vi "PID_controller_15.vi"() -> ()   [LabVIEW 2011]
panel:
  out "do_tune":bool
  in  "Tune":bool
  out "Temp Set Point (torr)":dbl
  in  "stop":bool
  out "fit":cluster{"element":dbl, "Value":dbl}[](array[cluster])
  out "err_avg":dbl
  out "Setpoint":string
  in  "Ks":dbl
  out "dt(s)":dbl
  out "windup error":dbl
  out "tPrev":dbl
  out "target value":dbl
  out "error(t-t0)":cluster{dbl, "Value":dbl}[](array[cluster])
  out "error":dbl
  out "tStart(s)":dbl
  out "S00":dbl
  out "S10":dbl
  out "S20":dbl
  out "S11":dbl
  out "S01":dbl
  out "weight":dbl[](array[numeric])
  in  "# of points to watch":i32
  in  "tSmooth(s)":dbl=-1.0
  out "t0":dbl
  out "error(t)":cluster{dbl, "Value":dbl}[](array[cluster])
  out "error out":errorcluster
  out "first":bool=TRUE
  out "XY Graph":T1(graph)
  out "current value":dbl
  in  "Period (s)":dbl
  out "dValue":dbl
  out "derivative":dbl
  out "integral":dbl
  out "Angle (deg)":dbl
  in  "Kd":dbl
  in  "Ki":dbl
  in  "Kp":dbl
  out "Current P (torr)":dbl
  in  "Set Point (torr)":dbl
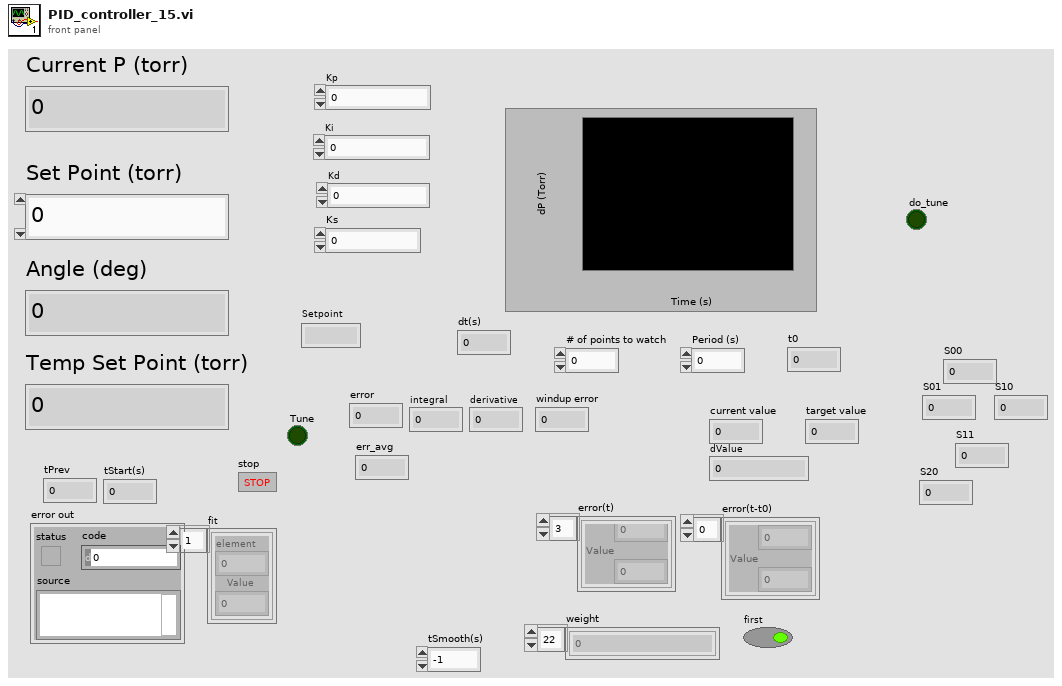
[diagram p1: front panel]
types:
  T1 = cluster{"Value":cluster{"element":dbl, "Value":dbl}[]}[]
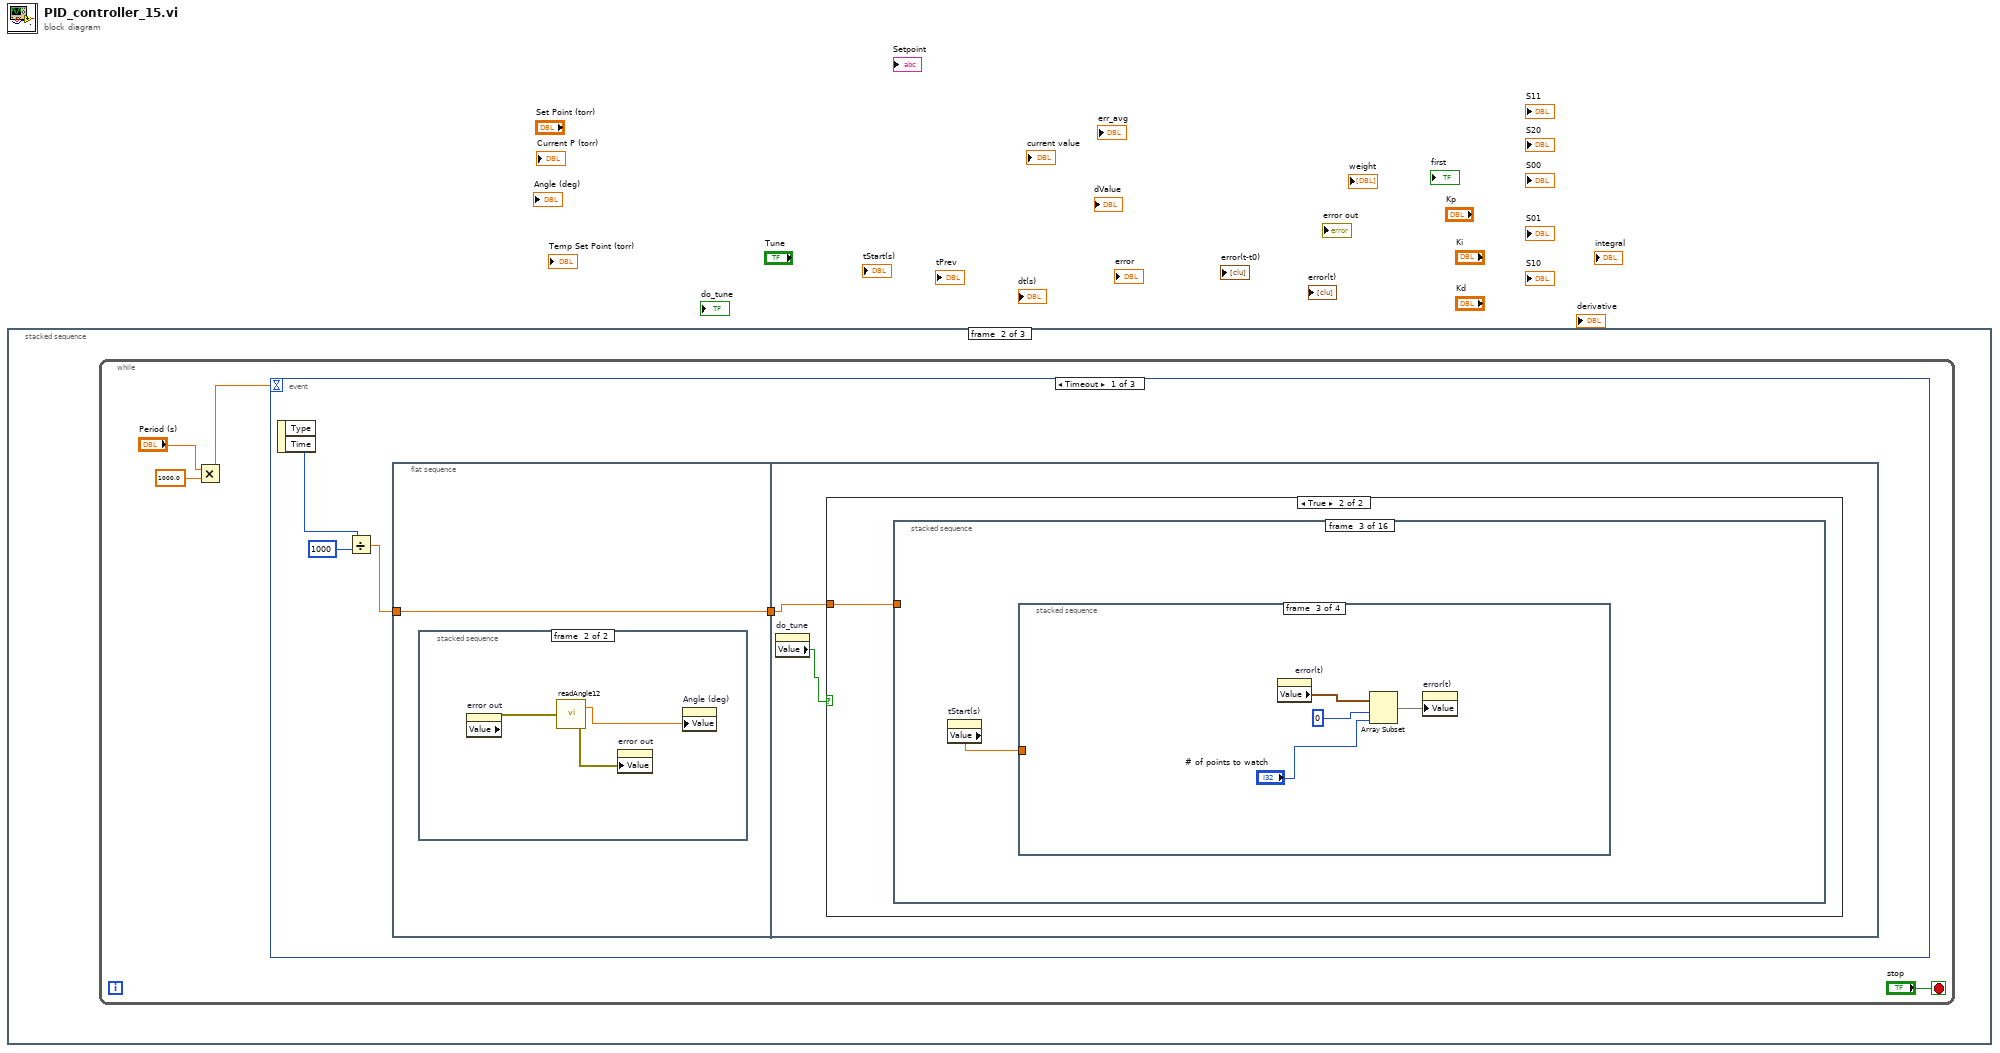
[diagram p0: block diagram]
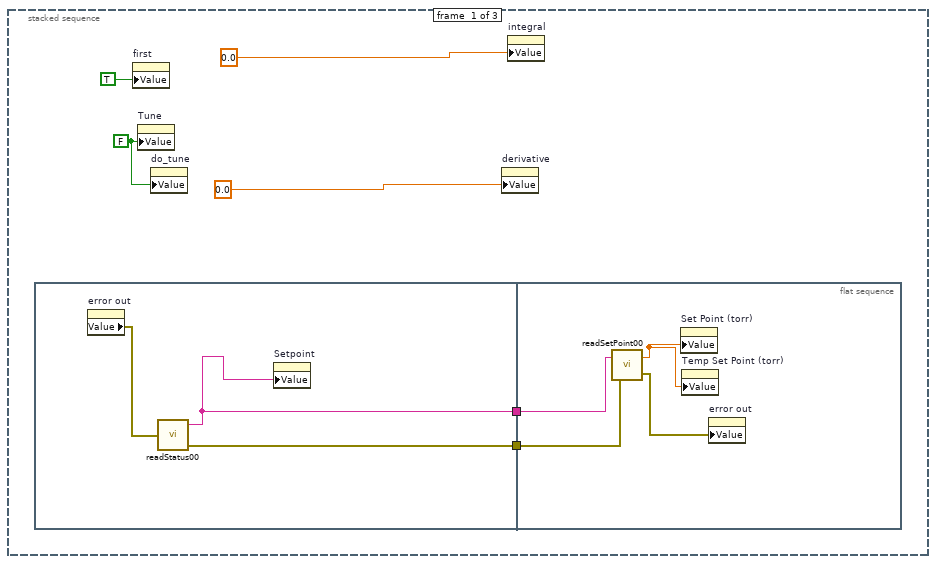
[diagram p2: hidden frame]
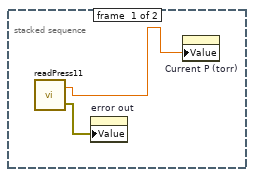
[diagram p3: hidden frame]
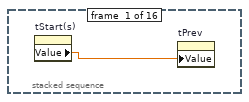
[diagram p5: hidden frame]
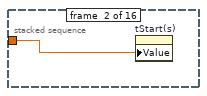
[diagram p6: hidden frame]
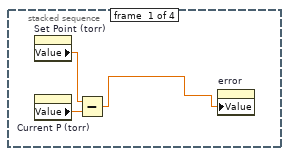
[diagram p7: hidden frame]
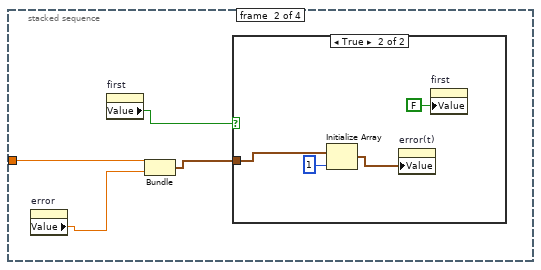
[diagram p8: hidden frame]
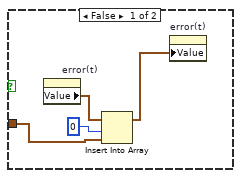
[diagram p9: hidden frame]
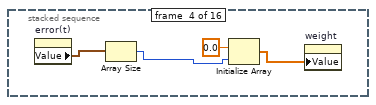
[diagram p11: hidden frame]
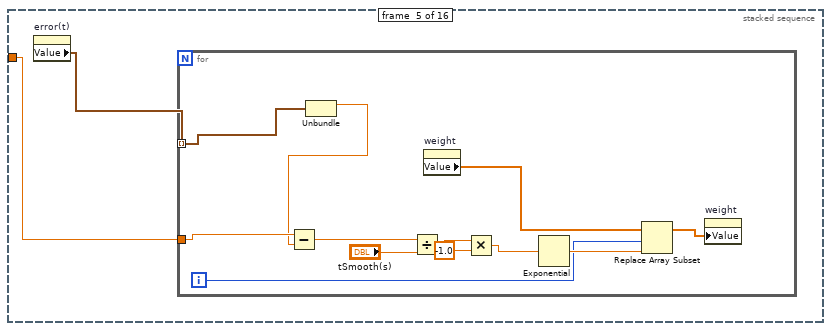
[diagram p12: hidden frame]
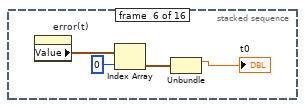
[diagram p13: hidden frame]
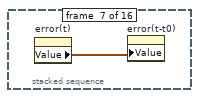
[diagram p14: hidden frame]
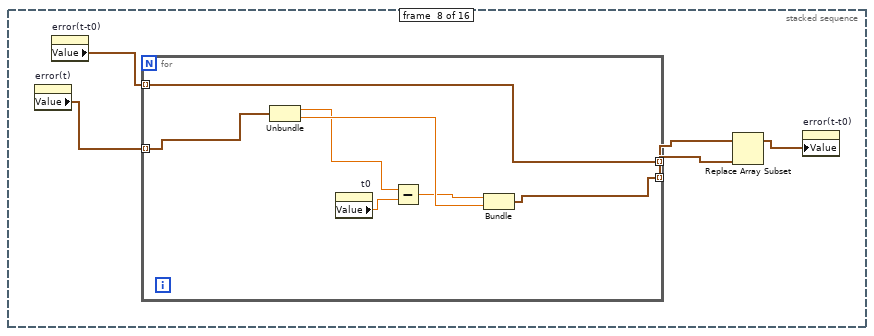
[diagram p15: hidden frame]
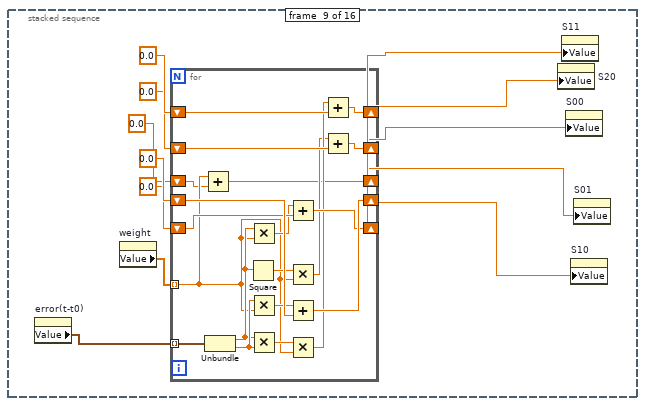
[diagram p16: hidden frame]
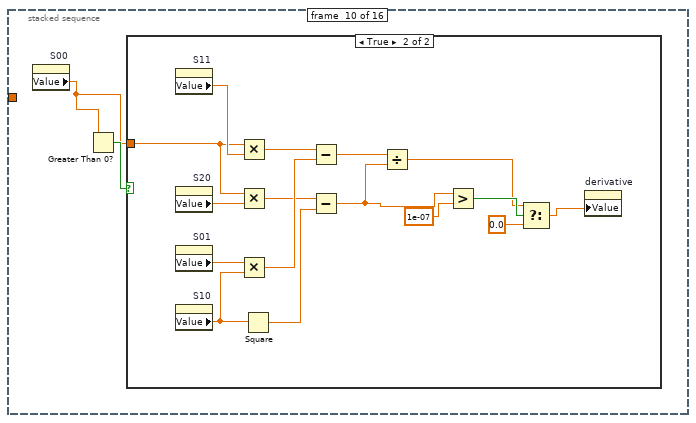
[diagram p17: hidden frame]
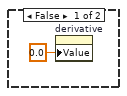
[diagram p18: hidden frame]
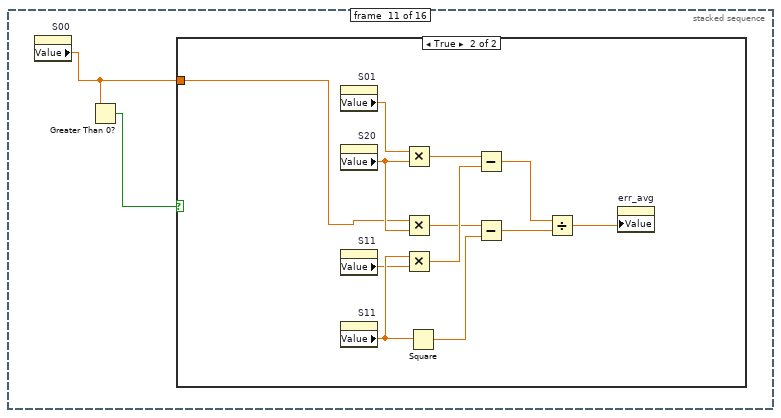
[diagram p19: hidden frame]
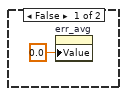
[diagram p20: hidden frame]
diagram:
  n1 = stacked-sequence {
    frame #0 {
      w1 = FALSE ("Tune")
      n2 = flat-sequence {
        tunnel: [w8] -> w3
        tunnel: [w7] -> w2
        tunnel: w3 -> [w13]
        tunnel: w2 -> [w12]
        frame #0 {
          n3 = property on="error out" class="Clust (strict)"() -> ("Value"=w9:errorcluster)  [unwired: 2 in, 2 out]
          n4 = call "readStatus00.vi"("error in"=w9) -> ("Setpoint"=w8:string, "error out"=w7:errorcluster)  [unwired: 1 out]
          n5 = property on="Setpoint" class="Str"("Value"=w8) -> ()  [unwired: 2 in, 2 out]
        }
        frame #1 {
          n6 = call "readSetPoint00.vi"("error in"=w12, "Setpoint"=w13) -> ("error out"=w11:errorcluster, "P"=w10:dbl)
          n7 = property on="Set Point (torr)" class="DigNum (strict)"("Value"=w10) -> ()  [unwired: 2 in, 2 out]
          n8 = property on="Temp Set Point (torr)" class="DigNum (strict)"("Value"=w10) -> ()  [unwired: 2 in, 2 out]
          n9 = property on="error out" class="Clust (strict)"("Value"=w11) -> ()  [unwired: 2 in, 2 out]
        }
      }
      n10 = property on="first" class="Bool (strict)"("Value"=TRUE ("first")) -> ()  [unwired: 2 in, 2 out]
      n11 = property on="Tune" class="Bool (strict)"("Value"=w1) -> ()  [unwired: 2 in, 2 out]
      n12 = property on="do_tune" class="Bool (strict)"("Value"=w1) -> ()  [unwired: 2 in, 2 out]
      n13 = property on="derivative" class="DigNum (strict)"("Value"=0.0 ("derivative")) -> ()  [unwired: 2 in, 2 out]
      n14 = property on="integral" class="DigNum (strict)"("Value"=0.0 ("integral")) -> ()  [unwired: 2 in, 2 out]
    }
    frame #1 {
      n15 = while {
        stop <- "stop" stop-if-true
        n16 = Multiply(x="Period (s)", y=1000.0) -> (x*y=w15:dbl)
        n17 = event shown="[0] Timeout" {
          selector: _ -> [_ _ _]
          dyn-events: _ -> [_ _ _]
          timeout: w15 -> [_ _ _]
          event Timeout {
            n18 = event-data() -> ("Time"=w21:u32)  [unwired: 1 in, 1 out]
            n19 = Divide(x=w21, y=u32 1000) -> (x/y=w19:dbl)
            n20 = flat-sequence {
              tunnel: w19 -> [w22]
              tunnel: [w22] -> w18
              tunnel: w18 -> [w29]
              frame #0 {
                n21 = stacked-sequence {
                  frame #0 {
                    n22 = call "readPress11.vi"() -> ("P"=w24:dbl, "error out"=w23:errorcluster)  [unwired: 1 in]
                    n23 = property on="error out" class="Clust (strict)"("Value"=w23) -> ()  [unwired: 2 in, 2 out]
                    n24 = property on="Current P (torr)" class="DigNum (strict)"("Value"=w24) -> ()  [unwired: 2 in, 2 out]
                  }
                  frame #1 {
                    n25 = property on="error out" class="Clust (strict)"() -> ("Value"=w26:errorcluster)  [unwired: 2 in, 2 out]
                    n26 = call "readAngle12.vi"("error in"=w26) -> ("angle"=w27:dbl, "error out"=w25:errorcluster)
                    n27 = property on="error out" class="Clust (strict)"("Value"=w25) -> ()  [unwired: 2 in, 2 out]
                    n28 = property on="Angle (deg)" class="DigNum (strict)"("Value"=w27) -> ()  [unwired: 2 in, 2 out]
                  }
                }
              }
              frame #1 {
                n29 = property on="do_tune" class="Bool (strict)"() -> ("Value"=w28:bool)  [unwired: 2 in, 2 out]
                n30 = case shown="True" w28 {
                  tunnel: w29 -> [_ w30]
                  frame False {
                  }
                  frame True {
                    n31 = stacked-sequence {
                      tunnel: w30 -> [_ w32 _ _ w57 _ _ _ _ _ _ _ _ _ _ _]
                      frame #0 {
                        n32 = property on="tStart(s)" class="DigNum (strict)"() -> ("Value"=w31:dbl)  [unwired: 2 in, 2 out]
                        n33 = property on="tPrev" class="DigNum (strict)"("Value"=w31) -> ()  [unwired: 2 in, 2 out]
                      }
                      frame #1 {
                        n34 = property on="tStart(s)" class="DigNum (strict)"("Value"=w32) -> ()  [unwired: 2 in, 2 out]
                      }
                      frame #2 {
                        n35 = property on="tStart(s)" class="DigNum (strict)"() -> ("Value"=w33:dbl)  [unwired: 2 in, 2 out]
                        n36 = stacked-sequence {
                          tunnel: w33 -> [_ w39 _ _]
                          frame #0 {
                            n37 = property on="Set Point (torr)" class="DigNum (strict)"() -> ("Value"=w35:dbl)  [unwired: 2 in, 2 out]
                            n38 = property on="Current P (torr)" class="DigNum (strict)"() -> ("Value"=w36:dbl)  [unwired: 2 in, 2 out]
                            n39 = Subtract(x=w35, y=w36) -> (x-y=w34:dbl)
                            n40 = property on="error" class="DigNum (strict)"("Value"=w34) -> ()  [unwired: 2 in, 2 out]
                          }
                          frame #1 {
                            n41 = property on="error" class="DigNum (strict)"() -> ("Value"=w37:dbl)  [unwired: 2 in, 2 out]
                            n42 = property on="first" class="Bool (strict)"() -> ("Value"=w40:bool)  [unwired: 2 in, 2 out]
                            n43 = Bundle("Value"=w39, "Value"=w37) -> (w38:cluster{"Value":dbl, "Value":dbl})  [unwired: 1 in]
                            n44 = case shown="True" w40 {
                              tunnel: w38 -> [w42 w47]
                              frame False {
                                n45 = property on="error(t)" class="Arr (strict)"() -> ("Value"=w43:cluster{dbl, "Value":dbl}[])  [unwired: 2 in, 2 out]
                                n46 = Insert Into Array(array=w43, index=0, new element=w42) -> (w41:cluster{dbl, "Value":dbl}[])
                                n47 = property on="error(t)" class="Arr (strict)"("Value"=w41) -> ()  [unwired: 2 in, 2 out]
                              }
                              frame True {
                                n48 = Initialize Array(w47, 1 ("dimension size")) -> (w45:cluster{"Value":dbl, "Value":dbl}[])
                                n49 = property on="error(t)" class="Arr (strict)"("Value"=w45) -> ()  [unwired: 2 in, 2 out]
                                n50 = property on="first" class="Bool (strict)"("Value"=FALSE ("first")) -> ()  [unwired: 2 in, 2 out]
                              }
                            }
                          }
                          frame #2 {
                            n51 = property on="error(t)" class="Arr (strict)"() -> ("Value"=w50:cluster{dbl, "Value":dbl}[])  [unwired: 2 in, 2 out]
                            n52 = Array Subset(array=w50, index=0, length="# of points to watch") -> (w52:cluster{dbl, "Value":dbl}[])
                            n53 = property on="error(t)" class="Arr (strict)"("Value"=w52) -> ()  [unwired: 2 in, 2 out]
                          }
                          frame #3 {
                          }
                        }
                      }
                      frame #3 {
                        n54 = property on="error(t)" class="Arr (strict)"() -> ("Value"=w56:cluster{dbl, "Value":dbl}[])  [unwired: 2 in, 2 out]
                        n55 = Array Size(array=w56) -> (size(s)=w54:i32)
                        n56 = Initialize Array(0.0 ("element"), w54) -> (w53:dbl[])
                        n57 = property on="weight" class="Arr (strict)"("Value"=w53) -> ()  [unwired: 2 in, 2 out]
                      }
                      frame #4 {
                        n58 = property on="error(t)" class="Arr (strict)"() -> ("Value"=w58:cluster{dbl, "Value":dbl}[])  [unwired: 2 in, 2 out]
                        n59 = for {
                          tunnel: w58 -> [w70] mode=indexing
                          tunnel: w57 -> [w69]
                          i -> [w65]
                          n60 = Unbundle(w70) -> (w68:dbl)  [unwired: 1 out]
                          n61 = Subtract(x=w69, y=w68) -> (x-y=w63:dbl)
                          n62 = Divide(x=w63, y="tSmooth(s)") -> (x/y=w61:dbl)
                          n63 = property on="weight" class="Arr (strict)"() -> ("Value"=w66:dbl[])  [unwired: 2 in, 2 out]
                          n64 = Multiply(x=w61, y=-1.0) -> (x*y=w59:dbl)
                          n65 = Exponential(1:w59) -> (0:w67:dbl)
                          n66 = Replace Array Subset(array=w66, new element=w67, index=w65) -> (w64:dbl[])
                          n67 = property on="weight" class="Arr (strict)"("Value"=w64) -> ()  [unwired: 2 in, 2 out]
                        }
                      }
                      frame #5 {
                        n68 = property on="error(t)" class="Arr (strict)"() -> ("Value"=w74:cluster{dbl, "Value":dbl}[])  [unwired: 2 in, 2 out]
                        n69 = Index Array(array=w74, index=0) -> (element=w72:cluster{dbl, "Value":dbl})
                        n70 = Unbundle(w72) -> (→"t0":dbl)  [unwired: 1 out]
                      }
                      frame #6 {
                        n71 = property on="error(t)" class="Arr (strict)"() -> ("Value"=w75:cluster{dbl, "Value":dbl}[])  [unwired: 2 in, 2 out]
                        n72 = property on="error(t-t0)" class="Arr (strict)"("Value"=w75) -> ()  [unwired: 2 in, 2 out]
                      }
                      frame #7 {
                        n73 = property on="error(t)" class="Arr (strict)"() -> ("Value"=w80:cluster{dbl, "Value":dbl}[])  [unwired: 2 in, 2 out]
                        n74 = property on="error(t-t0)" class="Arr (strict)"() -> ("Value"=w78:cluster{dbl, "Value":dbl}[])  [unwired: 2 in, 2 out]
                        n75 = for {
                          tunnel: w80 -> [w83] mode=indexing
                          tunnel: [w82] -> w79 mode=indexing
                          tunnel: w78 -> [w81] mode=indexing
                          tunnel: [w81] -> w77 mode=indexing
                          n76 = Unbundle(w83) -> (w84:dbl, "Value"=w86:dbl)
                          n77 = property on="t0" class="DigNum (strict)"() -> ("Value"=w87:dbl)  [unwired: 2 in, 2 out]
                          n78 = Subtract(x=w84, y=w87) -> (x-y=w85:dbl)
                          n79 = Bundle(w85, "Value"=w86) -> (w82:cluster{dbl, "Value":dbl})  [unwired: 1 in]
                        }
                        n80 = Replace Array Subset(array=w77, new element=w79) -> (w76:cluster{dbl, "Value":dbl}[])  [unwired: 1 in]
                        n81 = property on="error(t-t0)" class="Arr (strict)"("Value"=w76) -> ()  [unwired: 2 in, 2 out]
                      }
                      frame #8 {
                        n82 = property on="error(t-t0)" class="Arr (strict)"() -> ("Value"=w88:cluster{dbl, "Value":dbl}[])  [unwired: 2 in, 2 out]
                        n83 = property on="weight" class="Arr (strict)"() -> ("Value"=w95:dbl[])  [unwired: 2 in, 2 out]
                        n84 = for {
                          tunnel: w88 -> [w115] mode=indexing
                          shift-right: [w116] -> w90
                          shift-left: 0.0 -> [w119]
                          shift-right: [w112] -> w93
                          shift-left: 0.0 -> [w118]
                          shift-right: [w111] -> w92
                          shift-left: 0.0 -> [w117]
                          shift-right: [w113] -> w89
                          shift-left: 0.0 -> [w114]
                          tunnel: w95 -> [w102] mode=indexing
                          shift-right: [w100] -> w91
                          shift-left: 0.0 -> [w101]
                          n85 = Add(x=w102, y=w101) -> (x+y=w100:dbl)
                          n86 = Unbundle(w115) -> (w104:dbl, "Value"=w110:dbl)
                          n87 = Square(x=w104) -> (x^2=w106:dbl)
                          n88 = Multiply(x=w104, y=w102) -> (x*y=w103:dbl)
                          n89 = Multiply(x=w110, y=w102) -> (x*y=w109:dbl)
                          n90 = Multiply(x=w104, y=w110) -> (x*y=w108:dbl)
                          n91 = Add(x=w103, y=w114) -> (x+y=w113:dbl)
                          n92 = Multiply(x=w106, y=w102) -> (x*y=w105:dbl)
                          n93 = Add(x=w109, y=w119) -> (x+y=w116:dbl)
                          n94 = Multiply(x=w108, y=w102) -> (x*y=w107:dbl)
                          n95 = Add(x=w107, y=w118) -> (x+y=w112:dbl)
                          n96 = Add(x=w105, y=w117) -> (x+y=w111:dbl)
                        }
                        n97 = property on="S20" class="DigNum (strict)"("Value"=w92) -> ()  [unwired: 2 in, 2 out]
                        n98 = property on="S11" class="DigNum (strict)"("Value"=w93) -> ()  [unwired: 2 in, 2 out]
                        n99 = property on="S00" class="DigNum (strict)"("Value"=w91) -> ()  [unwired: 2 in, 2 out]
                        n100 = property on="S10" class="DigNum (strict)"("Value"=w89) -> ()  [unwired: 2 in, 2 out]
                        n101 = property on="S01" class="DigNum (strict)"("Value"=w90) -> ()  [unwired: 2 in, 2 out]
                      }
                      frame #9 {
                        n102 = property on="S00" class="DigNum (strict)"() -> ("Value"=w120:dbl)  [unwired: 2 in, 2 out]
                        n103 = Greater Than 0?(x=w120) -> (x > 0?=w121:bool)
                        n104 = case shown="True" w121 {
                          tunnel: w120 -> [_ w130]
                          frame False {
                            n105 = property on="derivative" class="DigNum (strict)"("Value"=0.0 ("derivative")) -> ()  [unwired: 2 in, 2 out]
                          }
                          frame True {
                            n106 = property on="S11" class="DigNum (strict)"() -> ("Value"=w132:dbl)  [unwired: 2 in, 2 out]
                            n107 = property on="S20" class="DigNum (strict)"() -> ("Value"=w131:dbl)  [unwired: 2 in, 2 out]
                            n108 = property on="S01" class="DigNum (strict)"() -> ("Value"=w129:dbl)  [unwired: 2 in, 2 out]
                            n109 = property on="S10" class="DigNum (strict)"() -> ("Value"=w133:dbl)  [unwired: 2 in, 2 out]
                            n110 = Multiply(x=w130, y=w132) -> (x*y=w138:dbl)
                            n111 = Multiply(x=w130, y=w131) -> (x*y=w136:dbl)
                            n112 = Multiply(x=w129, y=w133) -> (x*y=w137:dbl)
                            n113 = Square(x=w133) -> (x^2=w135:dbl)
                            n114 = Subtract(x=w138, y=w137) -> (x-y=w134:dbl)
                            n115 = Subtract(x=w136, y=w135) -> (x-y=w128:dbl)
                            n116 = Divide(x=w134, y=w128) -> (x/y=w124:dbl)
                            n117 = Greater?(x=w128, y=1e-07) -> (0:w126:bool)
                            n118 = Select(t=w124, s=w126, f=0.0) -> (s? t:f=w125:dbl)
                            n119 = property on="derivative" class="DigNum (strict)"("Value"=w125) -> ()  [unwired: 2 in, 2 out]
                          }
                        }
                      }
                      frame #10 {
                        n120 = property on="S00" class="DigNum (strict)"() -> ("Value"=w139:dbl)  [unwired: 2 in, 2 out]
                        n121 = Greater Than 0?(x=w139) -> (x > 0?=w140:bool)
                        n122 = case shown="True" w140 {
                          tunnel: w139 -> [_ w143]
                          frame False {
                            n123 = property on="err_avg" class="DigNum (strict)"("Value"=0.0 ("Pavg")) -> ()  [unwired: 2 in, 2 out]
                          }
                          frame True {
                            n124 = property on="S01" class="DigNum (strict)"() -> ("Value"=w144:dbl)  [unwired: 2 in, 2 out]
                            n125 = property on="S20" class="DigNum (strict)"() -> ("Value"=w147:dbl)  [unwired: 2 in, 2 out]
                            n126 = property on="S11" class="DigNum (strict)"() -> ("Value"=w145:dbl)  [unwired: 2 in, 2 out]
                            n127 = property on="S11" class="DigNum (strict)"() -> ("Value"=w146:dbl)  [unwired: 2 in, 2 out]
                            n128 = Multiply(x=w144, y=w147) -> (x*y=w152:dbl)
                            n129 = Multiply(x=w143, y=w147) -> (x*y=w149:dbl)
                            n130 = Multiply(x=w146, y=w145) -> (x*y=w153:dbl)
                            n131 = Square(x=w146) -> (x^2=w150:dbl)
                            n132 = Subtract(x=w152, y=w153) -> (x-y=w148:dbl)
                            n133 = Subtract(x=w149, y=w150) -> (x-y=w151:dbl)
                            n134 = Divide(x=w148, y=w151) -> (x/y=w142:dbl)
                            n135 = property on="err_avg" class="DigNum (strict)"("Value"=w142) -> ()  [unwired: 2 in, 2 out]
                          }
                        }
                      }
                      frame #11 {
                        n136 = property on="error(t-t0)" class="Arr (strict)"() -> ("Value"=w157:cluster{dbl, "Value":dbl}[])  [unwired: 2 in, 2 out]
                        n137 = Array Size(array=w157) -> (size(s)=w156:i32)
                        n138 = Greater?(x=w156, y=1) -> (0:w154:bool)
                        n139 = case shown="True" w154 {
                          frame False {
                          }
                          frame True {
                            n140 = property on="error(t-t0)" class="Arr (strict)"() -> ("Value"=w161:cluster{dbl, "Value":dbl}[])  [unwired: 2 in, 2 out]
                            n141 = Array Size(array=w161) -> (size(s)=w171:i32)
                            n142 = Index Array(array=w161, index=0) -> (element=w169:cluster{dbl, "Value":dbl})
                            n143 = Unbundle(w169) -> (w164:dbl)  [unwired: 1 out]
                            n144 = Decrement(x=w171) -> (x-1=w170:i32)
                            n145 = Index Array(array=w161, index=w170) -> (element=w168:cluster{dbl, "Value":dbl})
                            n146 = Unbundle(w168) -> (w162:dbl)  [unwired: 1 out]
                            n147 = property on="derivative" class="DigNum (strict)"() -> ("Value"=w167:dbl)  [unwired: 2 in, 2 out]
                            n148 = property on="error" class="DigNum (strict)"() -> ("Value"=w165:dbl)  [unwired: 2 in, 2 out]
                            n149 = Multiply(x=w162, y=w167) -> (x*y=w166:dbl)
                            n150 = Add(x=w165, y=w166) -> (x+y=w163:dbl)
                            n151 = Bundle(w164, "Value"=w165) -> (w160:cluster{dbl, "Value":dbl})  [unwired: 1 in]
                            n152 = Bundle(w162, w163) -> (w159:cluster{dbl, dbl})  [unwired: 1 in]
                            n153 = Build Array(w160, w159) -> (→"fit":cluster{dbl, "Value":dbl}[])
                          }
                        }
                      }
                      frame #12 {
                        n154 = property on="error" class="DigNum (strict)"() -> ("Value"=w177:dbl)  [unwired: 2 in, 2 out]
                        n155 = property on="tPrev" class="DigNum (strict)"() -> ("Value"=w178:dbl)  [unwired: 2 in, 2 out]
                        n156 = property on="tStart(s)" class="DigNum (strict)"() -> ("Value"=w179:dbl)  [unwired: 2 in, 2 out]
                        n157 = Subtract(x=w179, y=w178) -> (x-y=w173:dbl)
                        n158 = property on="dt(s)" class="DigNum (strict)"("Value"=w173) -> ()  [unwired: 2 in, 2 out]
                        n159 = property on="integral" class="DigNum (strict)"() -> ("Value"=w175:dbl)  [unwired: 2 in, 2 out]
                        n160 = Multiply(x=w177, y=w173) -> (x*y=w176:dbl)
                        n161 = Add(x=w176, y=w175) -> (x+y=w174:dbl)
                        n162 = property on="integral" class="DigNum (strict)"("Value"=w174) -> ()  [unwired: 2 in, 2 out]
                      }
                      frame #13 {
                        n163 = property on="error" class="DigNum (strict)"() -> ("Value"=w180:dbl)  [unwired: 2 in, 2 out]
                        n164 = property on="Kp" class="DigNum (strict)"() -> ("Value"=w190:dbl)  [unwired: 2 in, 2 out]
                        n165 = property on="integral" class="DigNum (strict)"() -> ("Value"=w188:dbl)  [unwired: 2 in, 2 out]
                        n166 = property on="derivative" class="DigNum (strict)"() -> ("Value"=w186:dbl)  [unwired: 2 in, 2 out]
                        n167 = property on="Ki" class="DigNum (strict)"() -> ("Value"=w189:dbl)  [unwired: 2 in, 2 out]
                        n168 = property on="Kd" class="DigNum (strict)"() -> ("Value"=w187:dbl)  [unwired: 2 in, 2 out]
                        n169 = Multiply(x=w187, y=w186) -> (x*y=w183:dbl)
                        n170 = Multiply(x=w189, y=w188) -> (x*y=w184:dbl)
                        n171 = Multiply(x=w190, y=w180) -> (x*y=w185:dbl)
                        n172 = Add(x=w185, y=w184) -> (x+y=w182:dbl)
                        n173 = Add(x=w182, y=w183) -> (x+y=w181:dbl)
                        n174 = property on="dValue" class="DigNum (strict)"("Value"=w181) -> ()  [unwired: 2 in, 2 out]
                      }
                      frame #14 {
                        w201 = 90.0 ("y")
                        n175 = property on="dValue" class="DigNum (strict)"() -> ("Value"=w208:dbl)  [unwired: 2 in, 2 out]
                        n176 = property on="current value" class="DigNum (strict)"() -> ("Value"=w209:dbl)  [unwired: 2 in, 2 out]
                        n177 = Add(x=w209, y=w208) -> (x+y=w193:dbl)
                        "target value" <- w193
                        n178 = Less Than 0?(x=w193) -> (x < 0?=w205:bool)
                        n179 = Select(t=0.0, s=w205, f=w193) -> (s? t:f=w202:dbl)
                        n180 = property on="Setpoint" class="Str"() -> ("Value"=w192:string)  [unwired: 2 in, 2 out]
                        n181 = property on="error out" class="Clust (strict)"() -> ("Value"=w207:errorcluster)  [unwired: 2 in, 2 out]
                        n182 = Greater?(x=w202, y=w201) -> (0:w203:bool)
                        n183 = Select(t=w201, s=w203, f=w202) -> (s? t:f=w191:dbl)
                        n184 = Subtract(x=w191, y=w193) -> (x-y=w200:dbl)
                        "windup error" <- w200
                        n185 = call "writeSetPoint_00.vi"("error in"=w207, "P (Torr)"=w191, "Setpoint"=w192) -> ("error out"=w206:errorcluster)
                        n186 = property on="dt(s)" class="DigNum (strict)"() -> ("Value"=w199:dbl)  [unwired: 2 in, 2 out]
                        n187 = property on="Temp Set Point (torr)" class="DigNum (strict)"("Value"=w191) -> ()  [unwired: 2 in, 2 out]
                        n188 = property on="current value" class="DigNum (strict)"("Value"=w191) -> ()  [unwired: 2 in, 2 out]
                        n189 = property on="error out" class="Clust (strict)"("Value"=w206) -> ()  [unwired: 2 in, 2 out]
                        n190 = Multiply(x=w200, y=w199) -> (x*y=w198:dbl)
                        n191 = property on="integral" class="DigNum (strict)"() -> ("Value"=w195:dbl)  [unwired: 2 in, 2 out]
                        n192 = Multiply(x="Ks", y=w198) -> (x*y=w196:dbl)
                        n193 = Add(x=w196, y=w195) -> (x+y=w194:dbl)
                        n194 = property on="integral" class="DigNum (strict)"("Value"=w194) -> ()  [unwired: 2 in, 2 out]
                      }
                      frame #15 {
                        n195 = property on="fit" class="Arr (strict)"() -> ("Value"=w212:cluster{"element":dbl, "Value":dbl}[])  [unwired: 2 in, 2 out]
                        n196 = property on="error(t-t0)" class="Arr (strict)"() -> ("Value"=w211:cluster{dbl, "Value":dbl}[])  [unwired: 2 in, 2 out]
                        n197 = Build Cluster Array(w211, w212) -> (→"XY Graph":T1)
                      }
                    }
                  }
                }
              }
            }
          }
          event "Tune": Value Change {
            n198 = event-data() -> ()  [unwired: 1 in, 5 out]
            n199 = property on="Tune" class="Bool (strict)"() -> ("Value"=w213:bool)  [unwired: 2 in, 2 out]
            n200 = property on="do_tune" class="Bool (strict)"("Value"=w213) -> ()  [unwired: 2 in, 2 out]
            n201 = case shown="True" w213 {
              frame False {
                n202 = property on="Set Point (torr)" class="DigNum (strict)"() -> ("Value"=w216:dbl)  [unwired: 2 in, 2 out]
                n203 = property on="Setpoint" class="Str"() -> ("Value"=w217:string)  [unwired: 2 in, 2 out]
                n204 = property on="error out" class="Clust (strict)"() -> ("Value"=w215:errorcluster)  [unwired: 2 in, 2 out]
                n205 = call "writeSetPoint_00.vi"("error in"=w215, "P (Torr)"=w216, "Setpoint"=w217) -> ("error out"=w214:errorcluster)
                n206 = property on="error out" class="Clust (strict)"("Value"=w214) -> ()  [unwired: 2 in, 2 out]
              }
              frame True {
                n207 = property on="error out" class="Clust (strict)"() -> ("Value"=w220:errorcluster)  [unwired: 2 in, 2 out]
                n208 = property on="Setpoint" class="Str"() -> ("Value"=w219:string)  [unwired: 2 in, 2 out]
                n209 = call "readSetPoint00.vi"("error in"=w220, "Setpoint"=w219) -> ("error out"=w221:errorcluster, "P"=w218:dbl)
                n210 = property on="Temp Set Point (torr)" class="DigNum (strict)"("Value"=w218) -> ()  [unwired: 2 in, 2 out]
                n211 = property on="Set Point (torr)" class="DigNum (strict)"("Value"=w218) -> ()  [unwired: 2 in, 2 out]
                n212 = property on="error out" class="Clust (strict)"("Value"=w221) -> ()  [unwired: 2 in, 2 out]
                n213 = property on="current value" class="DigNum (strict)"("Value"=w218) -> ()  [unwired: 2 in, 2 out]
              }
            }
          }
          event "Set Point (torr)": Value Change {
            n214 = event-data() -> ()  [unwired: 1 in, 5 out]
            n215 = property on="Set Point (torr)" class="DigNum (strict)"() -> ("Value"=w224:dbl)  [unwired: 2 in, 2 out]
            n216 = property on="Setpoint" class="Str"() -> ("Value"=w225:string)  [unwired: 2 in, 2 out]
            n217 = property on="error out" class="Clust (strict)"() -> ("Value"=w223:errorcluster)  [unwired: 2 in, 2 out]
            n218 = call "writeSetPoint_00.vi"("error in"=w223, "P (Torr)"=w224, "Setpoint"=w225) -> ("error out"=w222:errorcluster)
            n219 = property on="error out" class="Clust (strict)"("Value"=w222) -> ()  [unwired: 2 in, 2 out]
          }
        }
      }
    }
    frame #2 {
      n220 = disable-structure shown="Disabled" {
        frame Disabled {
          n221 = flat-sequence {
            frame #0 {
              n222 = call "WriteAdaptorr03.vi"("string to write"="D5") -> ()  [unwired: 1 in, 1 out]
            }
            frame #1 {
              n223 = property on="Setpoint" class="Str"() -> ("Value"=w228:string)  [unwired: 2 in, 2 out]
              n224 = Concatenate Strings("Press ", w228, " on AdapTorr") -> (w227:string)
              n225 = One Button Dialog(message=w227) -> ()  [unwired: 1 in, 1 out]
            }
          }
        }
        frame Enabled {
        }
      }
    }
  }
